vi "RT_TVA_READ.vi"(8 "error in (no error)":errorcluster, 11 "FPGA VI  IN":refnum<k20>) -> (0 "error out":errorcluster, 1 "Data":u64[](array[numeric]), 3 "FPGA VI  Out":refnum<k20>)   [LabVIEW 2017]
uses:
  <vilib>/Utility/error.llb/Error Cluster From Error Code.vi
  <vilib>/RVI Host/nirviSupport.llb/nirviErrorClusterFromErrorCode.vi
  <vilib>/rvi/errors/niLvFpgaAdjustHostInterfaceError.vi
  <vilib>/rvi/interface/nirviMethod/nirviMethod.xnode
  <vilib>/rvi/interface/nirviMethod/StockFPGA_InlinedMethodWaitForSingleIRQ.vi
  <vilib>/FPGAPlugInAG/Dynamic/niLvFpga_WaitOnIrq_Dynamic.vi
  <vilib>/FPGAPlugInAG/Dynamic/niLvFpga_ReadFifo_Dynamic.vi
  <vilib>/rvi/errors/niLvFpgaMergeErrorWithErrorCode.vi
  <vilib>/FPGAPlugInAG/Dynamic/niLvFpga_AcknowledgeIrq_Dynamic.vi
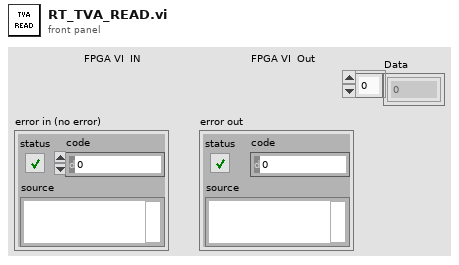
[diagram p1: front panel]
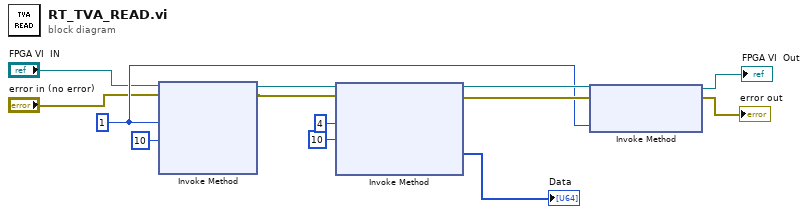
[diagram p0: block diagram]
diagram:
  w9 = 1 ("IRQ Number(s)")
  n1 = xnode "Invoke Method"("FPGA VI Reference In"="FPGA VI  IN", "error in"="error in (no error)", "IRQ Number(s)"=w9, "Timeout (ms)"=10) -> ("FPGA VI Reference Out"=w10:refnum<k20>, "error out"=w11:errorcluster)  [unwired: 2 out]
  n2 = xnode "Invoke Method"("FPGA VI Reference In"=w10, "error in"=w11, "Number of Elements"=u32 4, "Timeout (ms)"=10) -> ("FPGA VI Reference Out"=w12:refnum<k20>, "error out"=w13:errorcluster, "Data"=→"Data":u64[])  [unwired: 1 out]
  n3 = xnode "Invoke Method"("FPGA VI Reference In"=w12, "error in"=w13, "IRQ Number(s)"=w9) -> ("FPGA VI Reference Out"=→"FPGA VI  Out":refnum<k20>, "error out"=→"error out":errorcluster)
